vi "getCamerasPositionByID.vi"(10 "Lado":enum16{"Esquerdo", "Direito"}(ring) caption="Enum", 11 "Field Size 2":T1) -> (3 "Cameras Positions":dbl[][](array[numeric]))   [LabVIEW 2018]
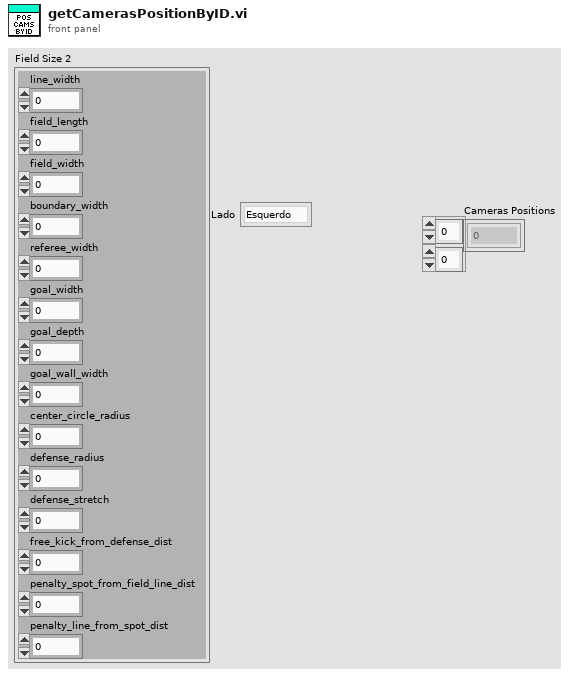
[diagram p1: front panel]
types:
  T1 = cluster{"line_width":u32, "field_length":u32, "field_width":u32, "boundary_width":u32, "referee_width":u32, "goal_width":u32, "goal_depth":u32, "goal_wall_width":u32, "center_circle_radius":u32, "defense_radius":u32, "defense_stretch":u32, "free_kick_from_defense_dist":u32, "penalty_spot_from_field_line_dist":u32, "penalty_line_from_spot_dist":u32}
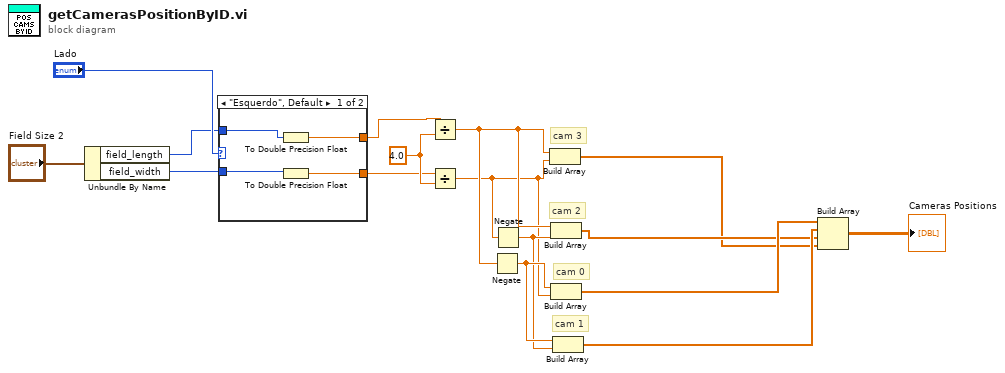
[diagram p0: block diagram]
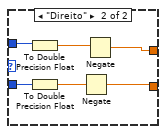
[diagram p2: hidden frame]
diagram:
  w15 = 4.0 ("y")
  # "cam 1"
  # "cam 0"
  # "cam 2"
  # "cam 3"
  n1 = Unbundle By Name("Field Size 2") -> ("field_length"=w2:u32, "field_width"=w4:u32)
  n2 = case shown="\"Esquerdo\", Default" "Lado" {
    tunnel: w4 -> [w20 w26]
    tunnel: [w19 w21] -> w3
    tunnel: w2 -> [w18 w25]
    tunnel: [w17 w23] -> w1
    frame "Esquerdo", Default {
      n3 = To Double Precision Float(number=w18) -> (double precision float=w17:dbl)
      n4 = To Double Precision Float(number=w20) -> (double precision float=w19:dbl)
    }
    frame "Direito" {
      n5 = To Double Precision Float(number=w25) -> (double precision float=w24:dbl)
      n6 = To Double Precision Float(number=w26) -> (double precision float=w22:dbl)
      n7 = Negate(x=w22) -> (-x=w21:dbl)
      n8 = Negate(x=w24) -> (-x=w23:dbl)
    }
  }
  n9 = Divide(x=w1, y=w15) -> (x/y=w13:dbl)
  n10 = Divide(x=w3, y=w15) -> (x/y=w11:dbl)
  n11 = Negate(x=w13) -> (-x=w14:dbl)
  n12 = Negate(x=w11) -> (-x=w12:dbl)
  n13 = Build Array(w13, w11) -> (w7:dbl[])
  n14 = Build Array(w13, w12) -> (w8:dbl[])
  n15 = Build Array(w14, w11) -> (w10:dbl[])
  n16 = Build Array(w14, w12) -> (w9:dbl[])
  n17 = Build Array(w10, w9, w8, w7) -> (→"Cameras Positions":dbl[][])
